vi "加标仪器启动命令 (子VI).vi"(8 "错误输入（无错误）":errorcluster, 10 "启动命令":enum16{"启动水样流程", "启动加标流程", "排液", "停止", "柱塞泵启动"}(ring), 11 "仪器":enum16{"", "氨氮", "总磷", "总氮", "CODMn", "CODCr"}(ring)=enum."氨氮") -> (0 "错误输出":errorcluster)   [LabVIEW 2016, in "质控单元.lvlib"]
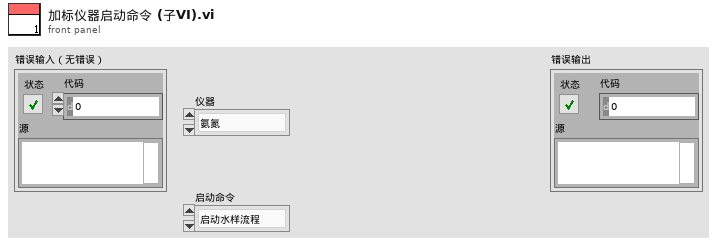
[diagram p1: front panel]
types:
  T1 = cluster{"仪器":enum16{"", "氨氮", "总磷", "总氮", "CODMn", "CODCr"}, "starting address":u16, "value":u16}
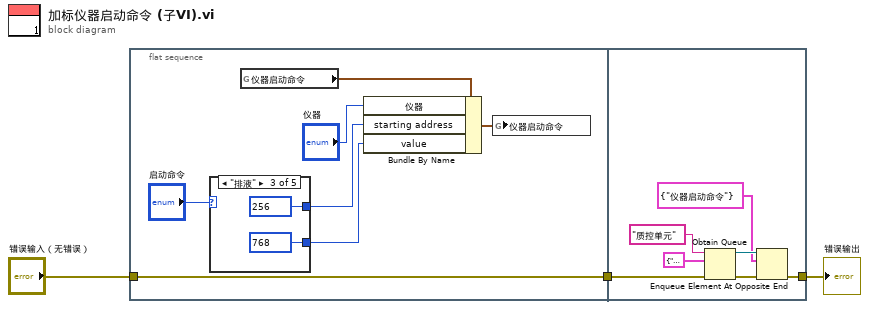
[diagram p0: block diagram]
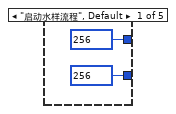
[diagram p2: hidden frame]
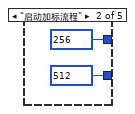
[diagram p3: hidden frame]
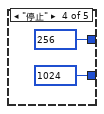
[diagram p4: hidden frame]
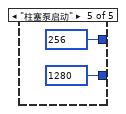
[diagram p5: hidden frame]
diagram:
  n1 = flat-sequence {
    tunnel: "错误输入（无错误）" -> [w7]
    tunnel: [w7] -> w2
    tunnel: w2 -> [w22]
    tunnel: [w21] -> w1
    frame #0 {
      n2 = case shown="\"排液\"" "启动命令" {
        tunnel: [u16 256 ("starting address") u16 256 ("starting address") u16 256 ("starting address") u16 256 ("starting address") u16 256 ("starting address")] -> w5
        tunnel: [u16 256 ("starting address") u16 512 ("starting address") u16 768 ("starting address") u16 1024 ("starting address") u16 1280 ("starting address")] -> w4
        frame "启动水样流程", Default {
        }
        frame "启动加标流程" {
        }
        frame "排液" {
        }
        frame "停止" {
        }
        frame "柱塞泵启动" {
        }
      }
      n3 = global read "质控内部交互全局.vi" "仪器启动命令"() -> (w8:T1)
      n4 = Bundle By Name(cluster=w8, "仪器"="仪器", "starting address"=w5, "value"=w4) -> (w9:T1)
      n5 = global write "质控内部交互全局.vi" "仪器启动命令"(w9) -> ()
    }
    frame #1 {
      n6 = Obtain Queue(name (unnamed)="质控单元" ("名称（未命名）"), element data type=cluster{"命令":string} {"命令"="启用模块"} ("元素"), error in (no error)=w22) -> (queue out=w25:refnum<queue>, error out=w24:errorcluster)  [unwired: 2 in, 1 out]
      n7 = Enqueue Element At Opposite End(queue=w25, element=cluster{"命令":string} {"命令"="仪器启动命令"} ("元素"), error in (no error)=w24) -> (error out=w21:errorcluster)  [unwired: 1 in, 2 out]
    }
  }
  "错误输出" <- w1
